vi "Template - Scope Edge Triggered Acquisition.vi"() -> ()   [LabVIEW 2013]
doc: "This example shows how to configure the oscilloscope to perform an edge-triggered waveform acquisition."
uses:
  <instrlib>/_Template - Scope/Public/Data/Read Waveform (Single).vi
  <instrlib>/_Template - Scope/Template - Scope.lvlib
panel:
  in  "Time per Division (0.0005 s)":dbl=0.0005
  in  "Serial Configuration":T1={"Baud Rate"=9600, "Parity"=0, "Data Bits"=7, "Stop Bits"=10, "Flow Control"=0} {"Flow Control" items=["None", "XON/XOFF", "RTS/CTS", "XON/XOFF & RTS/CTS", "DTR/DSR", "XON/XOFF & DTR/DSR"]; "Stop Bits" items=["1.0"=10, "1.5"=15, "2.0"=20]; "Data Bits" items=["7"=7, "8"=8]; "Parity" items=["None", "Odd", "Even", "Mark", "Space"]; "Baud Rate" items=["300"=300, "600"=600, "1200"=1200, "2400"=2400, "4800"=4800, "9600"=9600, "19200"=19200]}
  in  "Vertical Coupling (1: DC)":u16(ring)=1 items=["AC", "DC", "Ground"]
  in  "Probe Attenuation (1.0)":dbl=1.0
  in  "Vertical Range (1.0 V)":dbl=1.0
  in  "Trigger Level (0.0 V)":dbl
  out "Waveform Data":waveform(dbl)(graph)
  in  "Channel (1: Channel 1)":u16(ring)=1 items=["Channel 1"=1, "Channel 2"=2]
  in  "VISA resource name":refnum<visa-resource-name>
  # "(c) 2007 <Enter Company Name Here>.  ALL RIGHTS RESERVED."
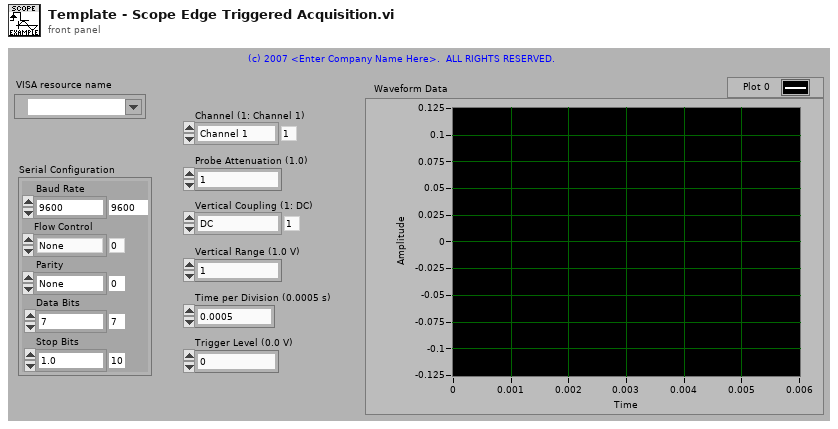
[diagram p1: front panel]
types:
  T1 = cluster{"Baud Rate":u32, "Parity":u16, "Data Bits":u16, "Stop Bits":u16, "Flow Control":u16}
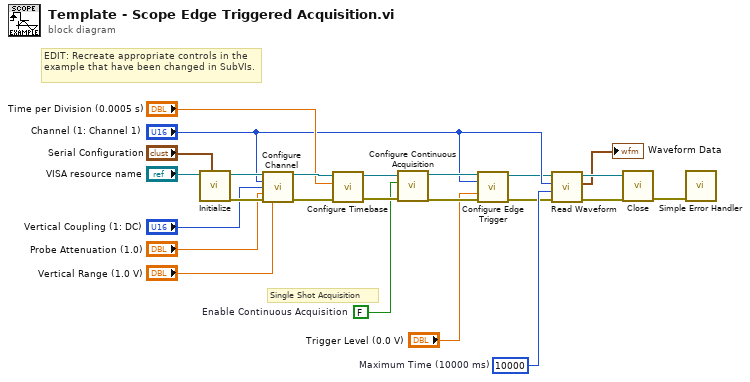
[diagram p0: block diagram]
diagram:
  w2 = u32 10000  # Maximum Time (10000 ms)
  w12 = FALSE  # Enable Continuous Acquisition
  # "EDIT: Recreate appropriate controls in the example that have been changed in SubVIs."
  # "Single Shot Acquisition"
  n1 = call <instrlib>:"Initialize.vi"("Serial Configuration"="Serial Configuration", "VISA resource name"="VISA resource name") -> ("error out"=w19:errorcluster, "VISA resource name out"=w20:refnum<visa-resource-name>)  [unwired: 8 in]
  n2 = call <instrlib>:"Configure Channel.vi"("VISA resource name"=w20, "Channel (1: Channel 1)"="Channel (1: Channel 1)", "Vertical Coupling (1: DC)"="Vertical Coupling (1: DC)", "Probe Attenuation (1.0)"="Probe Attenuation (1.0)", "error in (no error)"=w19, "Vertical Range (10.0 V)"="Vertical Range (1.0 V)") -> ("VISA resource name out"=w22:refnum<visa-resource-name>, "error out"=w23:errorcluster)  [unwired: 8 in]
  n3 = call <instrlib>:"Configure Timebase.vi"("error in (no error)"=w23, "Time per Division (0.0005 s)"="Time per Division (0.0005 s)", "VISA resource name"=w22) -> ("error out"=w15:errorcluster, "VISA resource name out"=w18:refnum<visa-resource-name>)  [unwired: 7 in]
  n4 = call <instrlib>:"Configure Continuous Acquisition.vi"("error in (no error)"=w15, "Enable Continuous Acquisition (T:Enable)"=w12, "VISA resource name"=w18) -> ("error out"=w16:errorcluster, "VISA resource name out"=w17:refnum<visa-resource-name>)  [unwired: 7 in]
  n5 = call <instrlib>:"Configure Edge Trigger.vi"("VISA resource name"=w17, "Trigger Source (1: Channel 1)"="Channel (1: Channel 1)", "Trigger Level (0.0 V)"="Trigger Level (0.0 V)", "error in (no error)"=w16) -> ("VISA resource name out"=w3:refnum<visa-resource-name>, "error out"=w1:errorcluster)  [unwired: 10 in]
  n6 = call-poly <instrlib>:"Read Waveform.vi"("error in (no error)"=w1, "Maximum Time (10000 ms)"=w2, "Channel (1: Channel 1)"="Channel (1: Channel 1)", "VISA resource name"=w3) -> ("error out"=w5:errorcluster, "Waveform Data"=→"Waveform Data":waveform(dbl), "VISA resource name out"=w7:refnum<visa-resource-name>)  [unwired: 5 in]
  n7 = call <instrlib>:"Close.vi"("error in (no error)"=w5, "VISA resource name"=w7) -> ("error out"=w24:errorcluster)  [unwired: 9 in]
  n8 = call <vilib>:"Simple Error Handler.vi"("error in (no error)"=w24) -> ()  [unwired: 4 in, 5 out]
